vi "PPSSelfTest.vi"(8 "error in":errorcluster, 11 "IT-M6018C in":refnum<class "IT-M6018C.lvclass">) -> (0 "error out":errorcluster, 2 "Self-Test Result Message":string, 3 "IT-M6018C out":refnum<class "IT-M6018C.lvclass">)   [LabVIEW 2023, in "HardwareAbstractionLayer_LVOOP.lvlib" / "IT-M6018C.lvclass"]
uses:
  IT-M6018C.lvclass
  PowerSupply.lvclass
  <instrlib>/IT6000C/IT6000C.lvlib
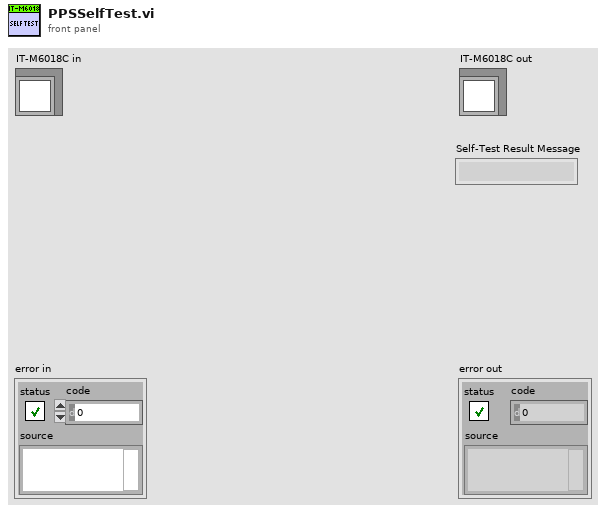
[diagram p1: front panel]
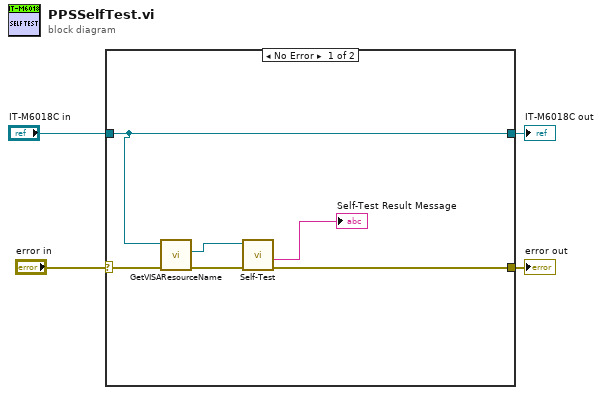
[diagram p0: block diagram]
diagram:
  n1 = case shown="No Error" "error in" {
    selector: "error in" -> [w10 w11]
    tunnel: [w7 w11] -> w3
    tunnel: "IT-M6018C in" -> [w9 w12]
    tunnel: [w9 w12] -> w1
    frame No Error {
      n2 = call "GetVISAResourceName.vi"("error in (no error)"=w10, "object in"=w9) -> ("error out"=w8:errorcluster, "VISA resource name"=w6:refnum<visa-resource-name>)  [unwired: 7 in, 1 out]
      n3 = call <instrlib>:"Self-Test.vi"("error in (no error)"=w8, "VISA resource name"=w6) -> ("error out"=w7:errorcluster, "Self-Test Result Message"=→"Self-Test Result Message":string)  [unwired: 6 in, 2 out]
    }
    frame Error {
    }
  }
  "error out" <- w3
  "IT-M6018C out" <- w1
